vi "Collide.vi"(8 "error in (no error)":errorcluster, 9 "CollideAll?":bool, 10 "Colliders":refnum<class "GameObject.lvclass">[](array[class]), 11 "Object in":refnum<class "GameObject.lvclass">) -> (0 "error out":errorcluster, 3 "Object out":refnum<class "GameObject.lvclass">)   [LabVIEW 2019, in "RT_Game.lvlib" / "GameObject.lvclass"]
uses:
  GameObject/GameObject.lvclass
  GameObject/GameObject.lvclass/GameObject.ctl
  Globals.vi
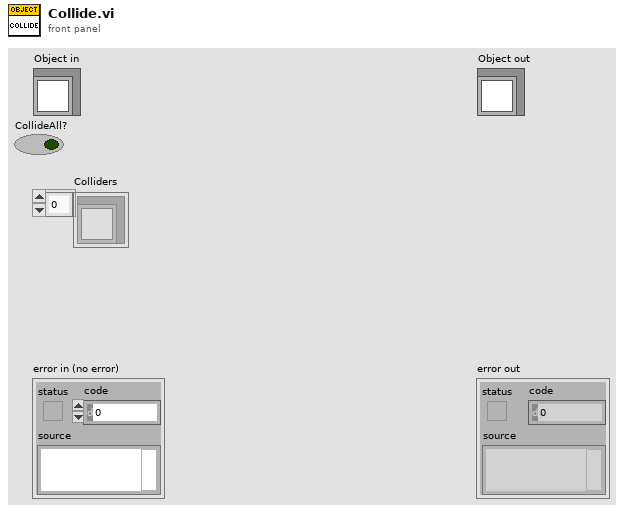
[diagram p1: front panel]
types:
  T1 = typedef "Velocity.ctl" = cluster{"x":dbl, "y":dbl}
  T2 = typedef "RT_Game.lvlib/Game.lvclass/Coordinate.ctl" = cluster{"x":dbl, "y":dbl}
  T3 = typedef "RT_Game.lvlib/Direction.ctl" = enum16{"none", "Both", "left", "right", "up", "down"}
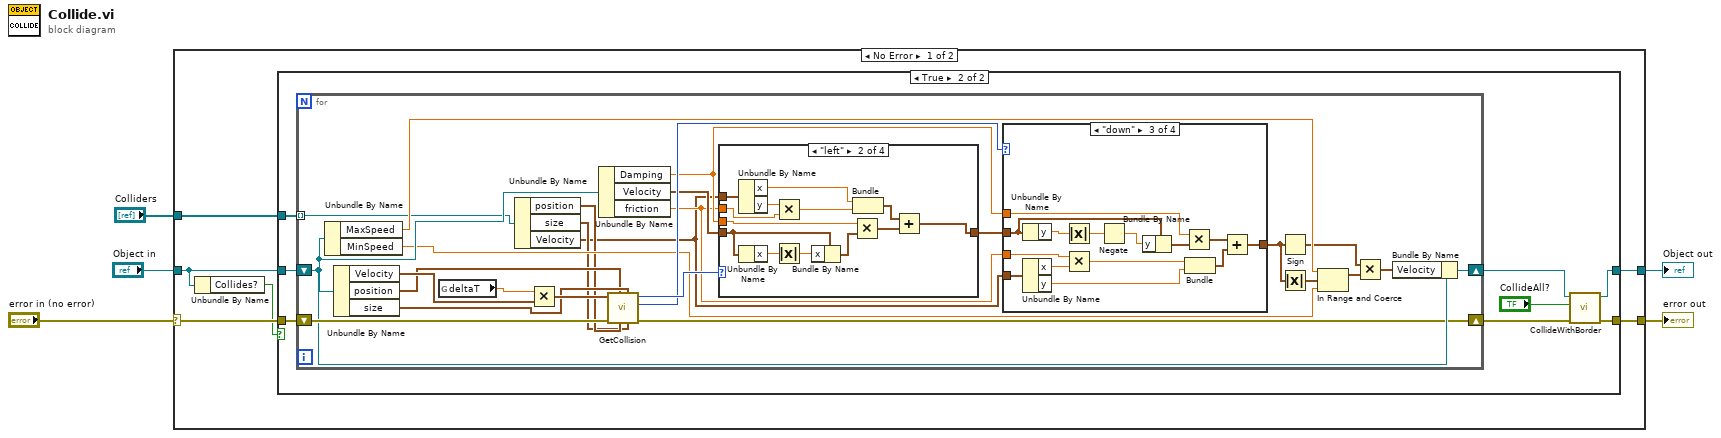
[diagram p0: block diagram]
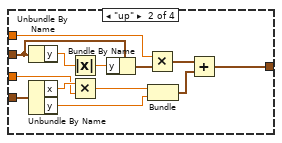
[diagram p4: hidden frame]
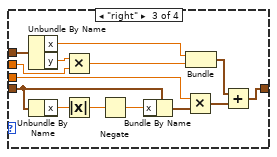
[diagram p7: hidden frame]
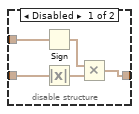
[diagram p9: hidden frame]
diagram:
  n1 = case shown="No Error" "error in (no error)" {
    selector: "error in (no error)" -> [w11 w115]
    tunnel: [w9 w115] -> w4
    tunnel: [w8 w114] -> w3
    tunnel: "Object in" -> [w7 w114]
    tunnel: "Colliders" -> [w10 _]
    frame No Error {
      n2 = Unbundle By Name(w7) -> ("Collides?"=w6:bool)
      n3 = case shown="True" w6 {
        tunnel: w11 -> [w12 w21]
        tunnel: w7 -> [w13 w19]
        tunnel: w10 -> [_ w18]
        tunnel: [w12 w17] -> w9
        tunnel: [w13 w15] -> w8
        frame False {
        }
        frame True {
          n4 = for {
            shift-right: [w43] -> w20
            shift-left: w21 -> [w47]
            shift-right: [w29] -> w16
            shift-left: w19 -> [w46]
            tunnel: w18 -> [w25] mode=indexing
            n5 = Unbundle By Name(w46) -> ("MaxSpeed"=w37:dbl, "MinSpeed"=w38:dbl)
            n6 = Unbundle By Name(w46) -> ("Velocity"=w45:T1, "position"=w26:T2, "size"=w27:T2)
            n7 = global read "Globals.vi" "deltaT"() -> (w44:dbl)
            n8 = Unbundle By Name(w25) -> ("position"=w24:T2, "size"=w23:T2, "Velocity"=w22:T1)
            n9 = Multiply(x=w44, y=w45) -> (x*y=w39:T1)
            n10 = Unbundle By Name(w46) -> ("Damping"=w32:dbl, "Velocity"=w40:T1, "friction"=w31:dbl)
            n11 = call "GetCollision.vi"("TheirSize"=w23, "MySize"=w27, "TheirPosition"=w24, "MyPosition"=w26, "error in (no error)"=w47, "Velocity"=w39) -> ("error out"=w43:errorcluster, "direction_y"=w41:T3, "direction_x"=w42:T3)  [unwired: 3 in]
            n12 = case shown="\"left\"" w42 {
              tunnel: w40 -> [w77 w86 w100 w107]
              tunnel: [w77 w88 w102 w106] -> w30
              tunnel: w22 -> [_ w90 w104 w105]
              tunnel: w32 -> [_ w82 w96 _]
              tunnel: w31 -> [_ w78 w91 _]
              frame "none", Default {
              }
              frame "left" {
                n13 = Unbundle By Name(w90) -> ("x"=w84:dbl, "y"=w80:dbl)
                n14 = Unbundle By Name(w86) -> ("x"=w85:dbl)
                n15 = Multiply(x=w80, y=w78) -> (x*y=w79:dbl)
                n16 = Absolute Value(x=w85) -> (abs(x)=w81:dbl)
                n17 = Bundle By Name(cluster=w86, "x"=w81) -> (w87:T1)
                n18 = Multiply(x=w82, y=w87) -> (x*y=w83:T1)
                n19 = Bundle("x"=w84, w79) -> (w89:cluster{"x":dbl, dbl})  [unwired: 1 in]
                n20 = Add(x=w89, y=w83) -> (x+y=w88:T1)
              }
              frame "right" {
                n21 = Unbundle By Name(w104) -> ("x"=w98:dbl, "y"=w93:dbl)
                n22 = Unbundle By Name(w100) -> ("x"=w99:dbl)
                n23 = Multiply(x=w93, y=w91) -> (x*y=w92:dbl)
                n24 = Absolute Value(x=w99) -> (abs(x)=w95:dbl)
                n25 = Negate(x=w95) -> (-x=w94:dbl)
                n26 = Bundle By Name(cluster=w100, "x"=w94) -> (w101:T1)
                n27 = Multiply(x=w96, y=w101) -> (x*y=w97:T1)
                n28 = Bundle("x"=w98, w92) -> (w103:cluster{"x":dbl, dbl})  [unwired: 1 in]
                n29 = Add(x=w103, y=w97) -> (x+y=w102:T1)
              }
              frame "Both" {
                n30 = disable-structure shown="Enabled" {
                  disable-tunnel: w107 -> [w112 w113]
                  disable-tunnel: [w111 w113] -> w106
                  disable-tunnel: w105 -> [w109 _]
                  frame Disabled {
                    n31 = Sign(1:w109) -> (0:w108:T1)
                    n32 = Absolute Value(x=w112) -> (abs(x)=w110:T1)
                    n33 = Multiply(x=w108, y=w110) -> (x*y=w111:T1)
                  }
                  frame Enabled {
                  }
                }
              }
            }
            n34 = case shown="\"down\"" w41 {
              tunnel: w30 -> [w48 w56 w70 w76]
              tunnel: [w48 w58 w72 w76] -> w34
              tunnel: w22 -> [_ w60 w74 _]
              tunnel: w32 -> [_ w52 w65 _]
              tunnel: w31 -> [_ w50 w62 _]
              frame "none", Default {
              }
              frame "up" {
                n35 = Unbundle By Name(w56) -> ("y"=w57:dbl)
                n36 = Unbundle By Name(w60) -> ("x"=w51:dbl, "y"=w59:dbl)
                n37 = Absolute Value(x=w57) -> (abs(x)=w53:dbl)
                n38 = Multiply(x=w51, y=w50) -> (x*y=w49:dbl)
                n39 = Bundle By Name(cluster=w56, "y"=w53) -> (w54:T1)
                n40 = Multiply(x=w52, y=w54) -> (x*y=w55:T1)
                n41 = Bundle(w49, "y"=w59) -> (w61:cluster{dbl, "y":dbl})  [unwired: 1 in]
                n42 = Add(x=w55, y=w61) -> (x+y=w58:T1)
              }
              frame "down" {
                n43 = Unbundle By Name(w70) -> ("y"=w71:dbl)
                n44 = Unbundle By Name(w74) -> ("x"=w64:dbl, "y"=w73:dbl)
                n45 = Absolute Value(x=w71) -> (abs(x)=w67:dbl)
                n46 = Multiply(x=w62, y=w64) -> (x*y=w63:dbl)
                n47 = Negate(x=w67) -> (-x=w66:dbl)
                n48 = Bundle By Name(cluster=w70, "y"=w66) -> (w68:T1)
                n49 = Multiply(x=w65, y=w68) -> (x*y=w69:T1)
                n50 = Bundle(w63, "y"=w73) -> (w75:cluster{dbl, "y":dbl})  [unwired: 1 in]
                n51 = Add(x=w69, y=w75) -> (x+y=w72:T1)
              }
              frame "Both" {
              }
            }
            n52 = Sign(1:w34) -> (0:w33:T1)
            n53 = Absolute Value(x=w34) -> (abs(x)=w35:T1)
            n54 = In Range and Coerce(upper limit=w37, x=w35, lower limit=w38) -> (coerced(x)=w36:T1)  [unwired: 1 out]
            n55 = Multiply(x=w33, y=w36) -> (x*y=w28:T1)
            n56 = Bundle By Name(cluster=w46, "Velocity"=w28) -> (w29:refnum<class "GameObject.lvclass">)
          }
          n57 = call "CollideWithBorder.vi"("error in (no error)"=w20, "CollideAll?"="CollideAll?", "Object in"=w16) -> ("error out"=w17:errorcluster, "Object out"=w15:refnum<class "GameObject.lvclass">)  [unwired: 7 in]
        }
      }
    }
    frame Error {
    }
  }
  "error out" <- w4
  "Object out" <- w3
